vi "Disabled.vi"(7 "Robot Mode":T2, 10 "Match Info":T1={"Autonomous Elapsed Seconds"=0.0, "TeleOp Elapsed Seconds"=0.0, "Disabled Elapsed Seconds"=0.0, "Visited Autonomous"=FALSE, "Visited TeleOp"=FALSE, "Visited Disabled"=FALSE, "Autonomous Settings"={"Autonomous Style"=enum."Independent", "VI Refnum"=refnum}}, 11 "Call Context":T3) -> ()   [LabVIEW 2015]
doc: "This VI is called each time a disabled packet is received from the DS. It is often used to prepare for the next robot mode, to calibrate sensors, etc."
uses:
  Robot Global Data.vi
  <vilib>/Rock Robotics/WPI/DriverStation/WPI_DriverStationRobotMode2.ctl
  <vilib>/Rock Robotics/WPI/DriverStation/WPI_DriverStationMatch Info.ctl
  <vilib>/Rock Robotics/WPI/DriverStation/WPI_DriverStationDerivedRobotMode.ctl
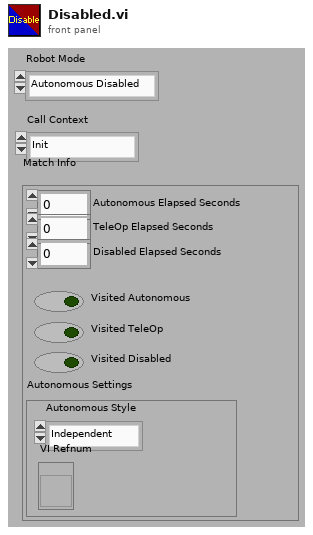
[diagram p1: front panel]
types:
  T1 = typedef "WPI_DriverStationMatch Info.ctl" = cluster{"Autonomous Elapsed Seconds":dbl, "TeleOp Elapsed Seconds":dbl, "Disabled Elapsed Seconds":dbl, "Visited Autonomous":bool, "Visited TeleOp":bool, "Visited Disabled":bool, "Autonomous Settings":cluster{"Autonomous Style":enum16{"Iterative", "Independent"}, "VI Refnum":refnum<vi>}}
  T2 = typedef "WPI_DriverStationRobotMode2.ctl" = enum16{"Autonomous Disabled", "Autonomous Enabled", "Teleop Disabled", "Teleop Enabled", "Disconnected", "Finish", "Test Disabled", "Test Enabled"}
  T3 = typedef "WPI_DriverStationDerivedRobotMode.ctl" = enum16{"Init", "Execute", "Stop"}
  T4 = typedef "TargetType.ctl" = enum16{"Not Hot", "Hot"}
  T5 = cluster{"Distance (ft)":dbl, "Target Center (-1 to 1)":cluster{"X":dbl, "Y":dbl}, "Left":bool, "State":T4, "Angle":dbl}
  T6 = typedef "WPI_GyroDevRef.ctl" = cluster{"DevStatus":errorcluster, "Analog Module":T7, "Analog Channel":T8, "Offset":dbl, "Gain (VoltsPerDegree/Second)":dbl}
  T7 = typedef "FPGA_TypedefAnalogModule.ctl" = enum16{"Analog Module 1", "Analog Module 2"}
  T8 = typedef "FPGA_AIChannel.ctl" = enum8{"AI 1", "AI 2", "AI 3", "AI 4", "AI 5", "AI 6", "AI 7", "AI 8", "Invalid"}
  T9 = enum16{"Queen", "King", "Rook", "Knight", "Pawn"}
  T10 = typedef "WPI_EncoderDevRef.ctl" = cluster{"DevStatus":errorcluster, "EncoderIndex":T11, "CounterIndex":T12, "DistancePerCount":dbl, "Decoding Type":T13}
  T11 = typedef "FPGA_EncoderIdx.ctl" = enum8{"Enc 0", "Enc 1", "Enc 2", "Enc 3", "Invalid"}
  T12 = typedef "FPGA_CounterCtrSystemIndex.ctl" = enum8{"Ctr 0", "Ctr 1", "Ctr 2", "Ctr 3", "Ctr 4", "Ctr 5", "Ctr 6", "Ctr 7", "Invalid"}
  T13 = typedef "WPI_EncoderType.ctl" = enum16{"1x", "2x", "4x"}
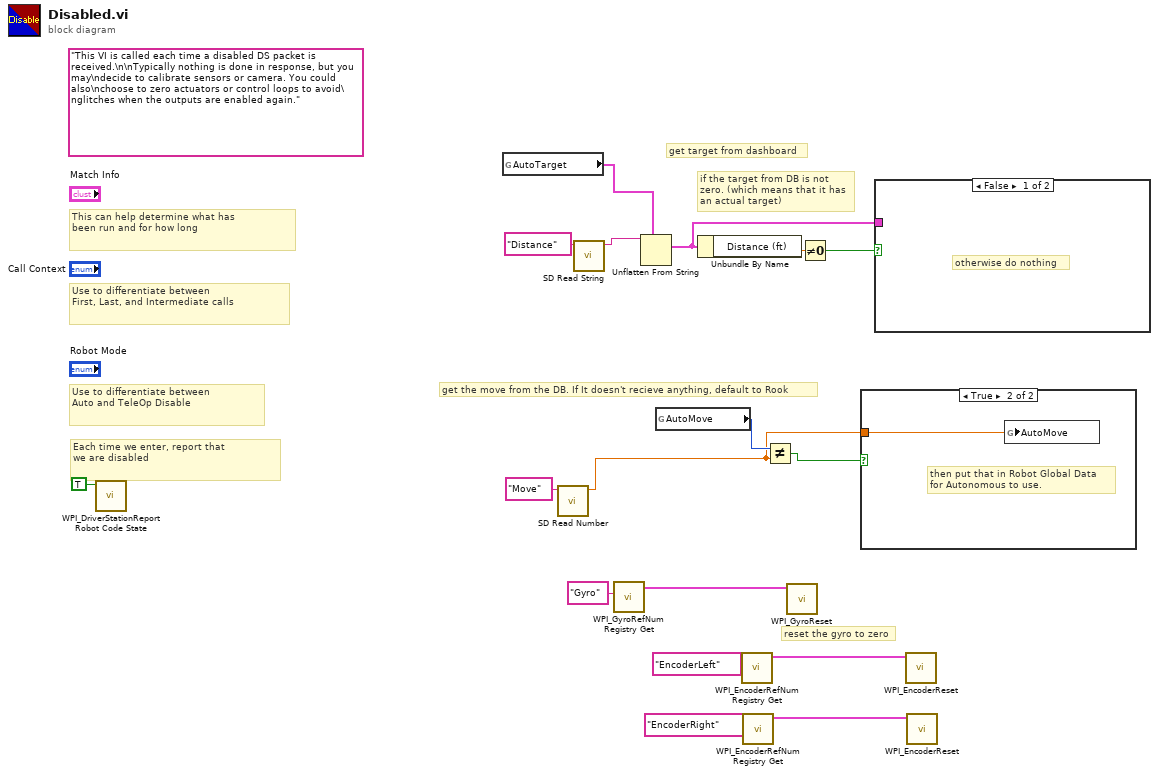
[diagram p0: block diagram]
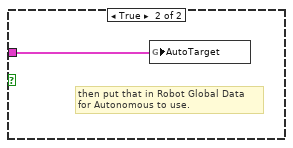
[diagram p3: hidden frame]
diagram:
  (unwired) "This VI is called each time a disabled DS packet is received.\n\nTypically nothing is done in response, but you may\ndecide to calibrate sensors or camera. You could also\nchoose to zero actuators or control loops to avoid\nglitches when the outputs are enabled again."
  # "get the move from the DB. If It doesn't recieve anything, default to Rook"
  # "reset the gyro to zero"
  # "if the target from DB is not\nzero. (which means that it has\nan actual target)"
  # "get target from dashboard"
  # "Each time we enter, report that\nwe are disabled"
  # "Use to differentiate between\nFirst, Last, and Intermediate calls"
  # "This can help determine what has\nbeen run and for how long"
  # "Use to differentiate between\nAuto and TeleOp Disable"
  n1 = call <vilib>:"WPI_DriverStationReport Robot Code State.vi"("Disabled"=TRUE ("Autonomous")) -> ()  [unwired: 10 in, 1 out]
  n2 = global read "Robot Global Data.vi" "AutoTarget"() -> (w12:T5)
  n3 = call <vilib>:"SD Read Number.vi"("Name"="Move") -> ("Numeric"=w1:dbl)  [unwired: 8 in, 2 out]
  n4 = call <vilib>:"SD Read String.vi"("Name"="Distance") -> ("String"=w13:string)  [unwired: 8 in, 2 out]
  n5 = call <vilib>:"WPI_GyroRefNum Registry Get.vi"("refnum name"="Gyro") -> ("GyroDevRef"=w15:T6)  [unwired: 9 in, 1 out]
  n6 = Unflatten From String(type=w12, binary string=w13) -> (value=w10:T5)  [unwired: 3 in, 2 out]
  n7 = global read "Robot Global Data.vi" "AutoMove"() -> (w2:T9)
  n8 = Unbundle By Name(w10) -> ("Distance (ft)"=w9:dbl)
  n9 = call <vilib>:"WPI_EncoderRefNum Registry Get.vi"("refnum name"="EncoderLeft") -> ("EncoderDevRef"=w8:T10)  [unwired: 9 in, 1 out]
  n10 = call <vilib>:"WPI_EncoderRefNum Registry Get.vi"("refnum name"="EncoderRight") -> ("EncoderDevRef"=w7:T10)  [unwired: 9 in, 1 out]
  n11 = Not Equal?(x=w2, y=w1) -> (x != y?=w3:bool)
  n12 = call <vilib>:"WPI_GyroReset.vi"("GyroDevRef"=w15) -> ()  [unwired: 9 in, 2 out]
  n13 = Not Equal To 0?(x=w9) -> (x != 0?=w11:bool)
  n14 = case shown="True" w3 {
    tunnel: w1 -> [_ w18]
    frame False {
      # "otherwise do nothing"
    }
    frame True {
      # "then put that in Robot Global Data \nfor Autonomous to use."
      n15 = global write "Robot Global Data.vi" "AutoMove"(w18) -> ()
    }
  }
  n16 = case shown="False" w11 {
    tunnel: w10 -> [_ w19]
    frame False {
      # "otherwise do nothing"
    }
    frame True {
      # "then put that in Robot Global Data \nfor Autonomous to use."
      n17 = global write "Robot Global Data.vi" "AutoTarget"(w19) -> ()
    }
  }
  n18 = call <vilib>:"WPI_EncoderReset.vi"("EncoderDevRef"=w8) -> ()  [unwired: 9 in, 2 out]
  n19 = call <vilib>:"WPI_EncoderReset.vi"("EncoderDevRef"=w7) -> ()  [unwired: 9 in, 2 out]
